vi "CreateObject.vi"(8 "error in (no error)":errorcluster) -> (0 "error out":errorcluster, 3 "DisplayWindow out":refnum<class "DisplayWindow.lvclass">)   [LabVIEW 2017, in "DisplayWindow.lvlib" / "DisplayWindow.lvclass"]
uses:
  DisplayWindow.lvclass
  DisplayWindow.lvclass/DisplayWindow.ctl
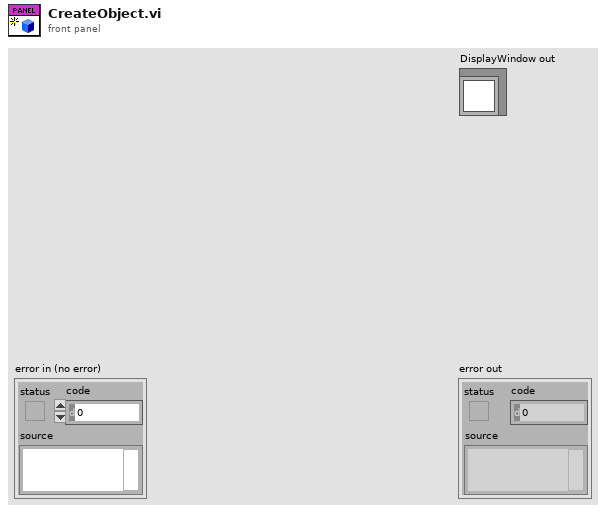
[diagram p1: front panel]
types:
  T1 = typedef "LVRectTypeDef.ctl" = cluster{"Left":i16, "Top":i16, "Right":i16, "Bottom":i16}
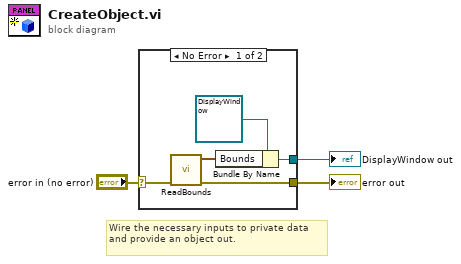
[diagram p0: block diagram]
diagram:
  # "Wire the necessary inputs to private data and provide an object out."
  n1 = case shown="No Error" "error in (no error)" {
    selector: "error in (no error)" -> [w5 w9]
    tunnel: [w4 w9] -> w2
    tunnel: [w7 _] -> w1
    frame No Error {
      n2 = call "ReadBounds.vi"("error in (no error)"=w5) -> ("error out"=w4:errorcluster, "Bounds"=w6:T1)  [unwired: 9 in]
      n3 = Bundle By Name(cluster=refnum<class "DisplayWindow.lvclass"> refnum ("DisplayWindow.lvlib:DisplayWindow.lvclass"), "Bounds"=w6) -> (w7:refnum<class "DisplayWindow.lvclass">)
    }
    frame Error {
    }
  }
  "error out" <- w2
  "DisplayWindow out" <- w1
